vi "control.vi"() -> ()   [LabVIEW 2010]
uses:
  <vilib>/sound2/lvsound2.llb/Sound Data Format.ctl
  <vilib>/addons/PixeLINK/Low Level Functions/CAMERA_FEATURES.llb/TDPU-CameraFeatures-PixelFormat.ctl
  <vilib>/sound2/lvsound2.llb/Sound Output Task ID.ctl
  <vilib>/vision/Image Controls.llb/IMAQ Image.ctl
panel:
  in  "Nueva Linea?":bool
  in  "Grabar":bool
  in  "Video?":bool
  in  "Compresion":u16(ring) items=["Emuzed H263 Video Encoder-DMO", "Emuzed H.264 Encoder-DMO", "Emuzed MPEG-4 SP Encoder-DMO", "DV Video Encoder", "MJPEG Compressor", "Cinepak Codec by Radius", "Intel IYUV codec", "Intel IYUV codec", "Microsoft RLE", "Microsoft Video 1"]
  out "Archivo de texto":path
  out "Selected Path for AVI":path
  out "time (ms)":u32
  out "Contraste":dbl(graph)
  out "Todo Funciona?":bool
  out "Waveform DAQ":waveform(dbl)(graph)
  out "Image":T1(plugin-control)
  in  "Tab Control":enum32{"DAQ", "Sound", "Camara", "Control"}(tab)
  in  "Calibracion DAQ":T2
  in  "DAQ Controls":T3={"Minimum Value"=-10.0, "Maximum Value"=10.0, "Physical Channel"="Dev1/ao0", "DAQ Fs (S/s)"=10000.0} {"Minimum Value" min=-10.0 max=0.0; "Maximum Value" min=0.0 max=10.0}
  in  "DAQ?":bool
  in  "Sound Controls":T5={"device ID"=0, "sound format"={"sample rate (S/s)"=44000.0, "number of channels"=2, "bits per sample"=16}, "time (ms)"=200.0}
  in  "Sound?":bool
  in  "Frecuencia":dbl
  in  "Selector":u16(ring) items=["776002034"]
  in  "Streeam?":bool
  out "Camara Funciona?":bool
  out "Contraste":dbl
  in  "Camera Parameters":T7 {"Pixel Format" items=["PIXEL_FORMAT_MONO8", "PIXEL_FORMAT_MONO16", "PIXEL_FORMAT_YUV422", "PIXEL_FORMAT_BAYER8_GRBG", "PIXEL_FORMAT_BAYER16_GRBG", "PIXEL_FORMAT_RGB24", "PIXEL_FORMAT_RGB48", "PIXEL_FORMAT_BAYER8_RGGB", "PIXEL_FORMAT_BAYER8_GBRG ", "PIXEL_FORMAT_BAYER8_BGGR ", "PIXEL_FORMAT_BAYER16_RGGB ", "PIXEL_FORMAT_BAYER16_GBRG", "PIXEL_FORMAT_BAYER16_BGGR", "PIXEL_FORMAT_RGB32"]}
  in  "Control Parameters":T8={"N Init Avg"=6, "N Avg Best"=3, "% Best to test"=0.95, "% Best to beat"=1.0}
  in  "lamda (nm)":dbl=546.1
  in  "Reset Control":bool
  in  "Control ON?":bool
  in  "Ajuste ON?":bool
  in  "stop":bool
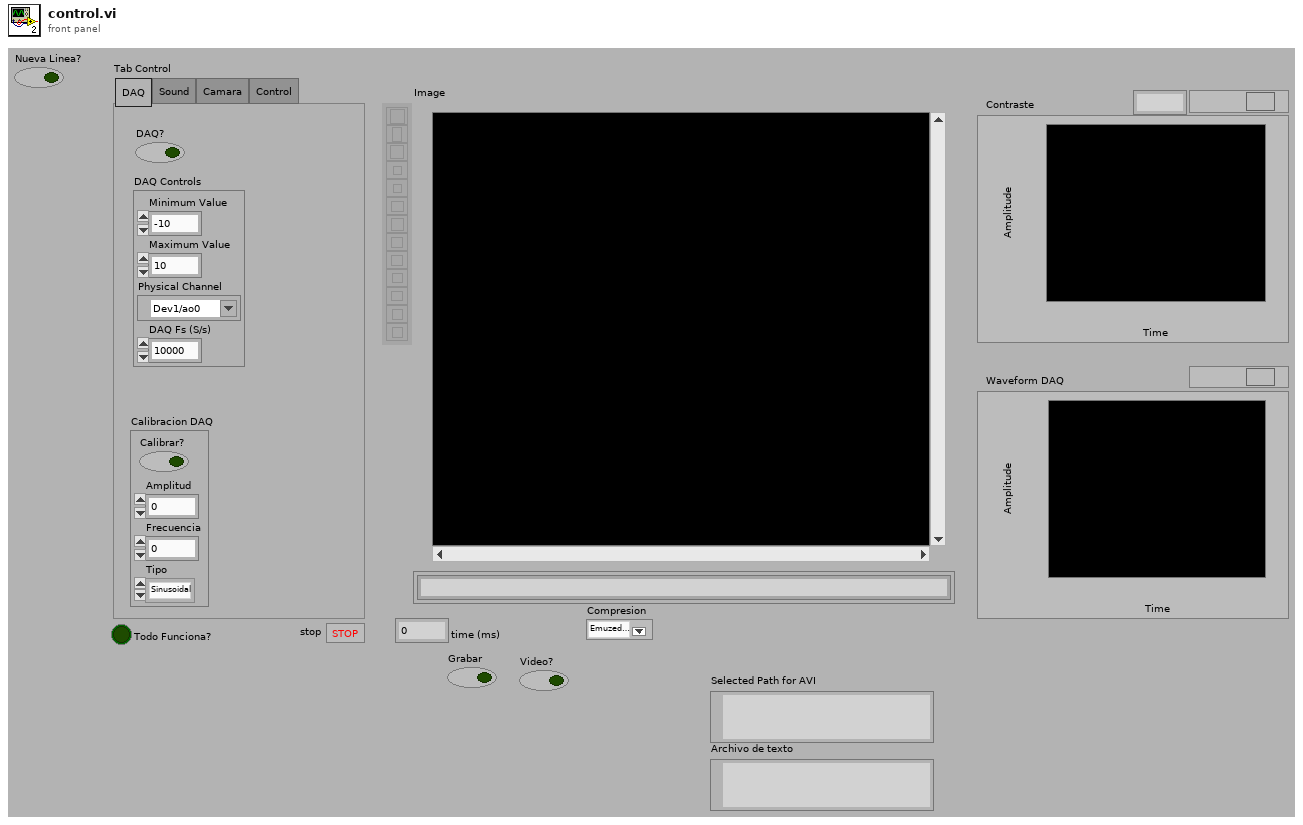
[diagram p1: front panel]
types:
  T1 = typedef "IMAQ Image.ctl" = refnum<image>
  T2 = cluster{"Calibrar?":bool, "Amplitud":dbl, "Frecuencia":dbl, "Tipo":enum16{"Sinusoidal", "Triangular", "Cuadrada"}}
  T3 = cluster{"Minimum Value":dbl, "Maximum Value":dbl, "Physical Channel":tag, "DAQ Fs (S/s)":dbl}
  T4 = typedef "Sound Data Format.ctl" = cluster{"sample rate (S/s)":dbl, "number of channels":i32, "bits per sample":i32}
  T5 = cluster{"device ID":u32, "sound format":T4, "time (ms)":dbl}
  T6 = typedef "TDPU-CameraFeatures-PixelFormat.ctl" = u16
  T7 = cluster{"Exposure Time (ms)":dbl, "Gain (dB)":dbl, "Saturation (%)":dbl, "Sharpness (%)":dbl, "Color Temperature":dbl, "ROI":cluster{"Top":i32, "Left":i32, "Width":i32, "Height":i32}, "White Balance Gain (dB)":cluster{"Red":dbl, "Green":dbl, "Blue":dbl}, "Gamma":dbl, "Pixel Format":T6, "FPS (frames/s)":i32}
  T8 = cluster{"N Init Avg":u32, "N Avg Best":u32, "% Best to test":dbl, "% Best to beat":dbl}
  T9 = cluster{"DAQ Fs (S/s)":dbl, "task":refnum<k21>, "error":errorcluster, "Min Value":dbl, "Max Value":dbl}
  T10 = cluster{"hCamera":u32, "Error":errorcluster, "uSerialNumber OUT":u32}
  T11 = typedef "Sound Output Task ID.ctl" = u32
  T12 = cluster{"task ID":T11, "error":errorcluster, "sound format":T4}
  T13 = cluster{"Amplitud":dbl, "Media":dbl, "Sigma":dbl}
  T14 = cluster{"hCamera":u32, "Error":errorcluster, "uSerialNumber":u32}
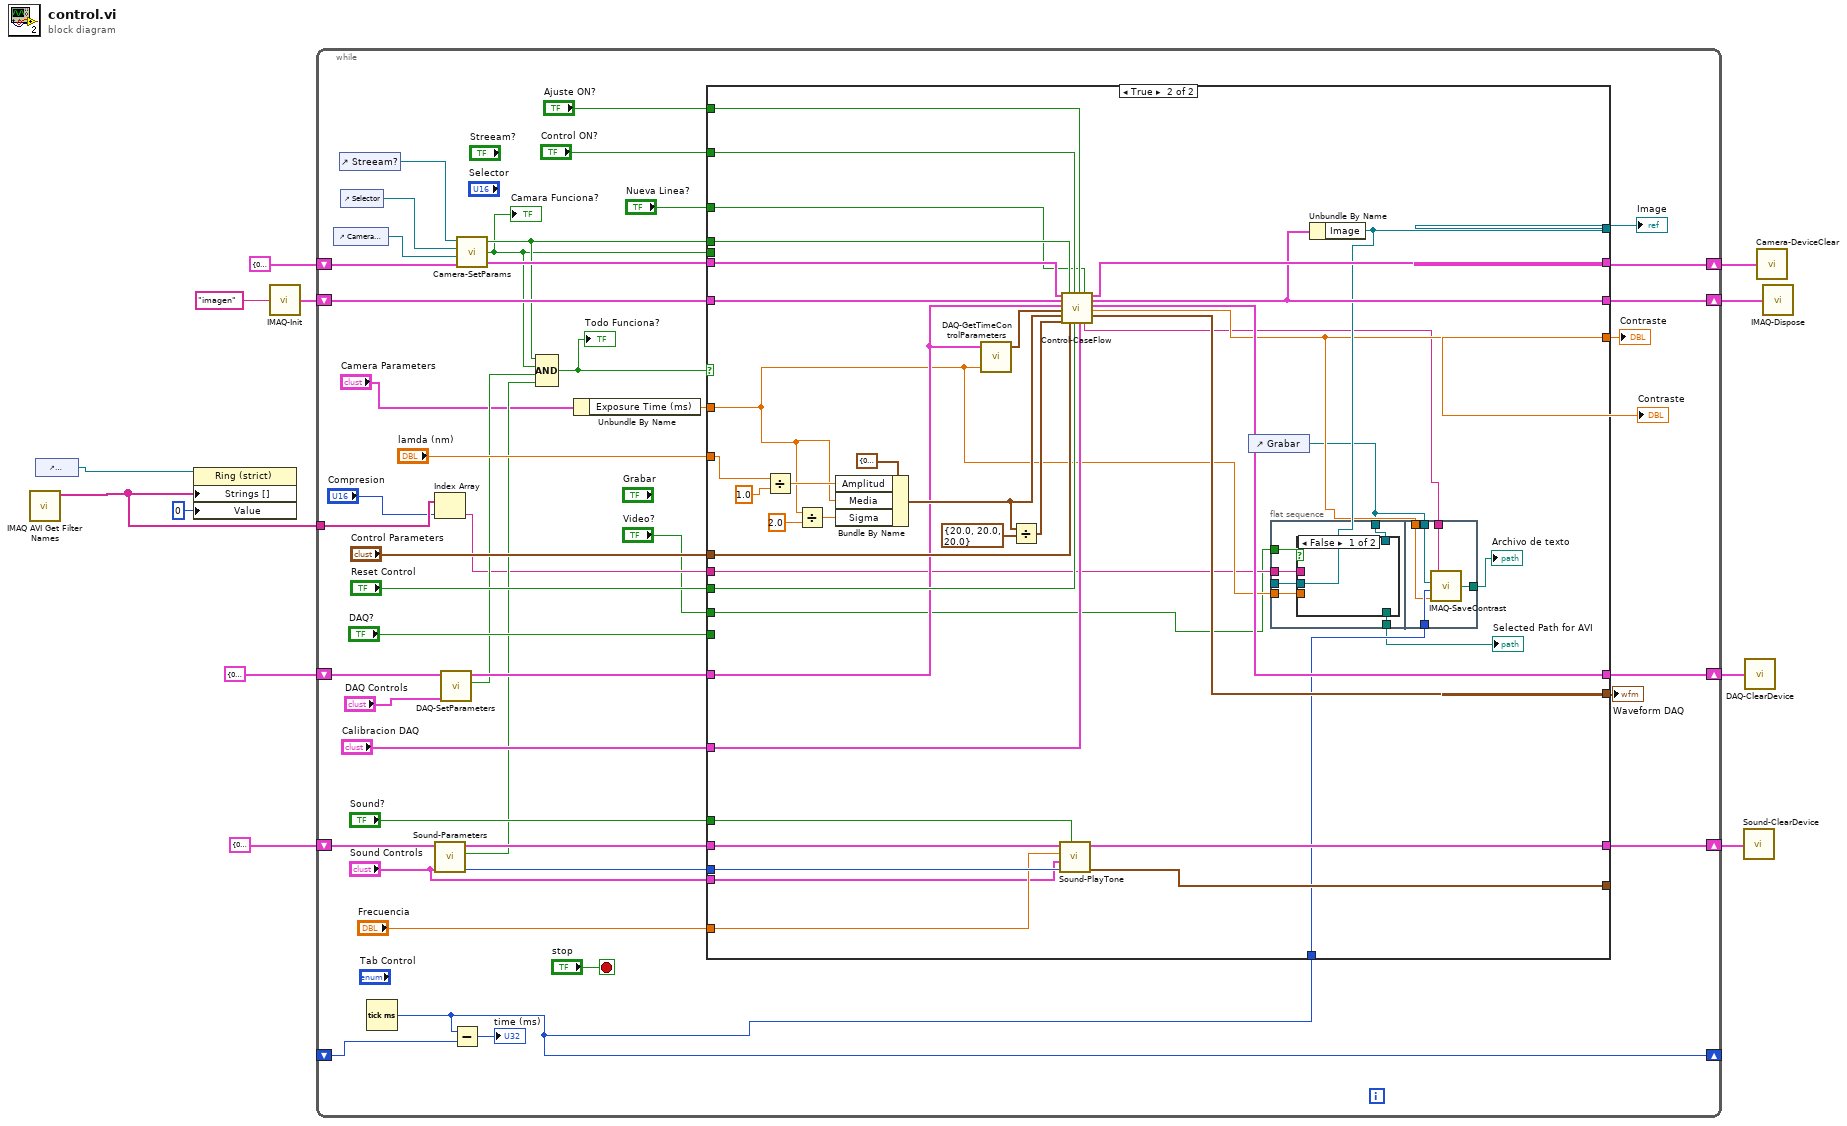
[diagram p0: block diagram]
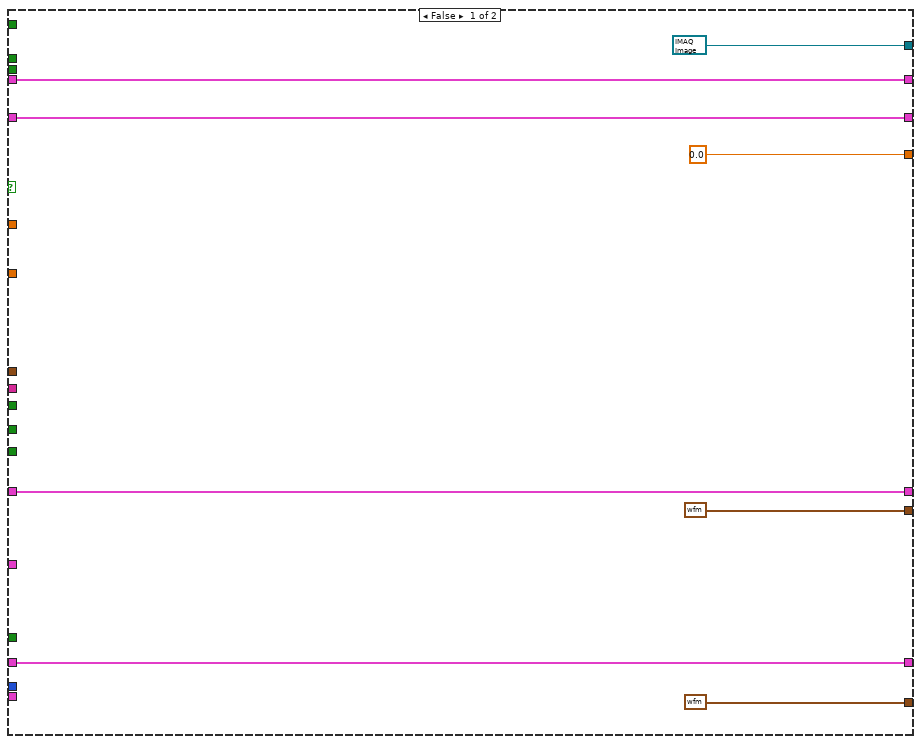
[diagram p2: hidden frame]
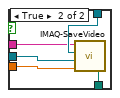
[diagram p3: hidden frame]
diagram:
  n1 = call "IMAQ AVI Get Filter Names"() -> ("Filter Names"=w2:string[])  [unwired: 10 in, 1 out]
  n2 = control-ref of="Compresion"() -> (w1:refnum<vi>)
  n3 = property on="Property Node" class="Ring (strict)"(reference=w1, "Strings []"=w2, "Value"=u16 0) -> ()  [unwired: 1 in, 2 out]
  n4 = call "IMAQ-Init.vi"("Image Name"="imagen") -> ("Image Device IN"=w8:cluster{"Image":T1, "errorImage":errorcluster})
  n5 = while {
    shift-right: [w50] -> w10
    shift-left: T9 {"DAQ Fs (S/s)"=0.0, "task"="", "error"={"status"=FALSE, "code"=0, "source"=""}, "Min Value"=0.0, "Max Value"=0.0} ("DAQ Device OUT") -> [w51]
    shift-right: [w47] -> w11
    shift-left: T12 {"task ID"=0, "error"={"status"=TRUE, "code"=0, "source"=""}, "sound format"={"sample rate (S/s)"=0.0, "number of channels"=0, "bits per sample"=0}} ("Sound Device OUT") -> [w46]
    shift-right: [w35] -> w5
    shift-left: w8 -> [w39]
    shift-right: [w38] -> w6
    shift-left: T10 {"hCamera"=0, "Error"={"status"=FALSE, "code"=0, "source"=""}, "uSerialNumber OUT"=0} ("Camera Device  IN") -> [w37]
    shift-right: [w20] -> _
    shift-left: _ -> [w22]
    tunnel: w2 -> [w19]
    stop <- "stop" stop-if-true
    n6 = control-ref of="Camera Parameters"() -> (w15:refnum<vi>)
    n7 = control-ref of="Streeam?"() -> (w41:refnum<vi>)
    n8 = control-ref of="Selector"() -> (w42:refnum<vi>)
    n9 = Tick Count (ms)() -> (millisecond timer value=w20:u32)
    n10 = Index Array(array=w19, index="Compresion") -> (element=w18:string)
    n11 = call "Sound-Parameters.vi"("Sound Controls"="Sound Controls", "Sound Device IN"=w46) -> ("#samples"=w48:u32, "En funcionamiento?"=w24:bool, "Sound Device OUT"=w49:T12)  [unwired: 3 in]
    n12 = call "DAQ-SetParameters.vi"("DAQ Controls"="DAQ Controls", "DAQ Device IN"=w51) -> ("En Funcionamiento?"=w25:bool, "DAQ Device OUT"=w55:T9)  [unwired: 4 in]
    n13 = Subtract(x=w20, y=w22) -> (x-y=→"time (ms)":u32)
    n14 = call "Camera-SetParams.vi"("Camera Device  IN"=w37, "Camera Parameters"=w15, "Selector"=w42, "Stream?"=w41) -> ("Camera Device OUT"=w40:T14, "Funciona?"=w26:bool, "Stream? OUT"=w27:bool)
    "Camara Funciona?" <- w26
    n15 = Compound Arithmetic op=AND(w27, w26, w25, w24) -> (w28:bool)
    "Todo Funciona?" <- w28
    n16 = Unbundle By Name("Camera Parameters") -> ("Exposure Time (ms)"=w31:dbl)
    n17 = case shown="True" w28 {
      tunnel: "DAQ?" -> [_ _]
      tunnel: w55 -> [w62 w83]
      tunnel: [waveform(dbl) {"t0"=timestamp(0 s since 1904-01-01), "dt"=1.0, "Y"=[]} ("Waveform") w77] -> w54
      tunnel: "Calibracion DAQ" -> [_ w84]
      tunnel: [w62 w96] -> w50
      tunnel: [waveform(dbl) {"t0"=timestamp(0 s since 1904-01-01), "dt"=1.0, "Y"=[]} ("Waveform") w106] -> _
      tunnel: w49 -> [w59 w105]
      tunnel: w48 -> [_ w104]
      tunnel: [w59 w103] -> w47
      tunnel: "Sound?" -> [_ w102]
      tunnel: "Frecuencia" -> [_ w101]
      tunnel: "Sound Controls" -> [_ w100]
      tunnel: w40 -> [w64 w99]
      tunnel: w39 -> [w63 w97]
      tunnel: [w64 w98] -> w38
      tunnel: [T1 refnum ("Image") w76] -> w36
      tunnel: [w63 w78] -> w35
      tunnel: [0.0 ("Contraste") w73] -> w23
      tunnel: w26 -> [_ _]
      tunnel: w27 -> [_ w81]
      tunnel: "lamda (nm)" -> [_ w89]
      tunnel: w31 -> [_ w75]
      tunnel: "Control Parameters" -> [_ w86]
      tunnel: "Reset Control" -> [_ w85]
      tunnel: "Ajuste ON?" -> [_ w80]
      tunnel: "Control ON?" -> [_ w79]
      tunnel: w20 -> [_ w74]
      tunnel: w18 -> [_ w70]
      tunnel: "Video?" -> [_ w68]
      tunnel: "Nueva Linea?" -> [_ w66]
      frame False {
      }
      frame True {
        n18 = Divide(x=w89, y=1.0) -> (x/y=w91:dbl)
        n19 = Divide(x=w75, y=2.0) -> (x/y=w94:dbl)
        n20 = Bundle By Name(cluster=T13 {"Amplitud"=0.0, "Media"=0.0, "Sigma"=0.0} ("Parametros Maximos"), "Amplitud"=w91, "Media"=w75, "Sigma"=w94) -> (w88:T13)
        n21 = call "DAQ-GetTimeControlParameters.vi"("tiempo (ms)"=w75, "DAQ Device IN"=w83) -> ("Time Control Parameters"=w95:cluster{"# samples":u32, "tiempos (ms)":dbl})  [unwired: 2 in, 1 out]
        n22 = Divide(x=w88, y=T13 {"Amplitud"=20.0, "Media"=20.0, "Sigma"=20.0}) -> (x/y=w87:T13)
        n23 = call "Sound-PlayTone.vi"("sound?"=w102, "# samples"=w104, "Sound Controls"=w100, "Frecuencia"=w101, "Sound Device IN"=w105) -> ("Waveform"=w106:waveform(dbl), "Sound Device OUT"=w103:T12)  [unwired: 3 in]
        n24 = call "Control-CaseFlow.vi"("Camera Device  IN"=w99, "Image Device IN"=w97, "DAQ Device IN"=w83, "Time Control Parameters"=w95, "Parametros Maximos"=w88, "detla Parametros"=w87, "Camara ON?"=w81, "Control Parameters"=w86, "Control?"=w79, "Reset Control"=w85, "Ajuste?"=w80, "Calibracion DAQ"=w84, "Nueva Linea?"=w66) -> ("Status Text"=w69:string, "Camera Device OUT"=w98:T10, "Image Device OUT"=w78:cluster{"Image":T1, "errorImage":errorcluster}, "DAQ Device OUT"=w96:T9, "Contraste"=w73:dbl, "Waveform"=w77:waveform(dbl))  [unwired: 1 out]
        n25 = control-ref of="Grabar"() -> (w67:refnum<vi>)
        n26 = flat-sequence {
          tunnel: w67 -> [w112]
          tunnel: w76 -> [w111]
          tunnel: w75 -> [w110]
          tunnel: [w109] -> w72
          tunnel: w70 -> [w108]
          tunnel: w68 -> [w107]
          tunnel: w67 -> [w122]
          tunnel: w74 -> [w121]
          tunnel: w73 -> [w120]
          tunnel: [w119] -> w71
          tunnel: w69 -> [w118]
          frame #0 {
            n27 = case shown="False" w107 {
              tunnel: w112 -> [_ w117]
              tunnel: w111 -> [_ w116]
              tunnel: w110 -> [_ w115]
              tunnel: [_ w114] -> w109
              tunnel: w108 -> [_ w113]
              frame False {
              }
              frame True {
                n28 = call "IMAQ-SaveVideo.vi"("Exposure Time (ms)"=w115, "Image"=w116, "Grabar"=w117, "Compression Filter"=w113) -> ("Selected Path for AVI"=w114:path)
              }
            }
          }
          frame #1 {
            n29 = call "IMAQ-SaveContrast.vi"("contraste"=w120, "tiempo (ms)"=w121, "Grabar"=w122, "Status"=w118) -> ("Archivo de texto"=w119:path)
          }
        }
        n30 = Unbundle By Name(w78) -> ("Image"=w76:T1)
        "Selected Path for AVI" <- w72
        "Archivo de texto" <- w71
      }
    }
    "Waveform DAQ" <- w54
    "Image" <- w36
    "Contraste" <- w23
    "Contraste" <- w23
  }
  n31 = call "Sound-ClearDevice.vi"("Sound Device OUT"=w11) -> ()
  n32 = call "DAQ-ClearDevice.vi"("DAQ Device IN"=w10) -> ()
  n33 = call "Camera-DeviceClear.vi"("Camera Device OUT"=w6) -> ()
  n34 = call "IMAQ-Dispose.vi"("Image Device IN"=w5) -> ()
